vi "ex_CheckEOF.vi"(2 "chunk in":string, 3 "file refs":T1) -> (0 "chunk remainder":string, 1 "EOF?":bool)   [LabVIEW 2020]
uses:
  <vilib>/express/express shared/ExFile.llb/ex_FileReference.ctl
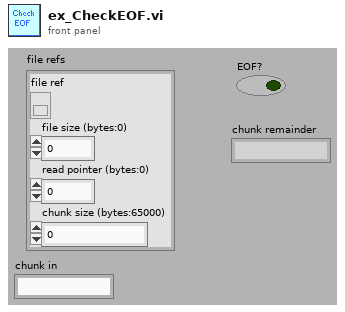
[diagram p1: front panel]
types:
  T1 = typedef "ex_FileReference.ctl" = cluster{"file ref":refnum<file>, "file size (bytes:0)":i32, "read pointer (bytes:0)":i32, "chunk size (bytes:65000)":i32}
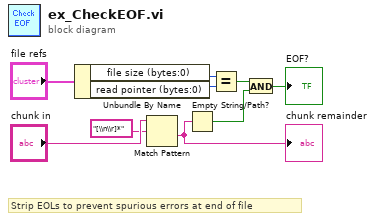
[diagram p0: block diagram]
diagram:
  # "Strip EOLs to prevent spurious errors at end of file"
  n1 = Unbundle By Name("file refs") -> ("file size (bytes:0)"=w5:i32, "read pointer (bytes:0)"=w4:i32)
  n2 = Match Pattern(string="chunk in", regular expression="[\\n\\r]*") -> (after substring=w2:string)  [unwired: 4 out]
  "chunk remainder" <- w2
  n3 = Empty String/Path?(string/path=w2) -> (empty?=w6:bool)
  n4 = Equal?(x=w5, y=w4) -> (x = y?=w7:bool)
  n5 = And(x=w7, y=w6) -> (x .and. y?=→"EOF?":bool)
